vi "Periodic - Drive PID Loop.vi"   [LabVIEW 2012]
uses:
  Globals/Jaguar Commands.vi
  Globals/Robot Jaguars.vi
  Globals/Encoders Global.vi
types:
  T1 = cluster{"proportional gain (Kc)":dbl, "integral time (Ti, min)":dbl, "derivative time (Td, min)":dbl}
  T2 = typedef "WPI_MotorControlDeviceRef.ctl" = cluster{"DeviceStatus":errorcluster, "Type":enum16{"PWM", "CAN"}, "PWM":cluster{"Digital Module":T3, "PWM Channel":T4, "DeadBand":T5}, "CAN":cluster{"Device Number":u8, "Control Mode":T6, "Semaphore":T7, "Max Vout":dbl}, "Invert":bool, "TransformRef":T8, "InvTransformRef":T8}
  T3 = typedef "FPGA_TypedefDigitalModule.ctl" = enum16{"Digital Module 1", "Digital Module 2"}
  T4 = typedef "FPGA_DIOPWMChannel.ctl" = enum8{"PWM 1", "PWM 2", "PWM 3", "PWM 4", "PWM 5", "PWM 6", "PWM 7", "PWM 8", "PWM 9", "PWM 10", "Invalid"}
  T5 = typedef "WPI_PWMDeadband.ctl" = cluster{"Name":string, "maxPositivePwm":i32, "minPositivePwm":i32, "centerPwm":i32, "maxNegativePwm":i32, "minNegativePwm":i32, "angularRange":u16}
  T6 = typedef "WPI_CANJaguar_ControlMode.ctl" = enum8{"Percent VBus", "Current", "Speed", "Position", "Voltage"}
  T7 = typedef "Semaphore RefNum" = refnum<k1>
  T8 = typedef "WPI_PWMTransform_ConPane.ctl" = refnum<vi>
  T9 = cluster{"Front Left Drive":T2, "Front Right Drive":T2, "Rear Left Drive":T2, "Rear Right Drive":T2, "Front Left Steer":T2, "Front Right Steer":T2, "Rear Left Steer":T2, "Rear Right Steer":T2}
  T10 = typedef "WPI_EncoderDevRef.ctl" = cluster{"DevStatus":errorcluster, "EncoderIndex":T11, "CounterIndex":T12, "DistancePerCount":dbl, "Decoding Type":T13}
  T11 = typedef "FPGA_EncoderIdx.ctl" = enum8{"Enc 0", "Enc 1", "Enc 2", "Enc 3", "Invalid"}
  T12 = typedef "FPGA_CounterCtrSystemIndex.ctl" = enum8{"Ctr 0", "Ctr 1", "Ctr 2", "Ctr 3", "Ctr 4", "Ctr 5", "Ctr 6", "Ctr 7", "Invalid"}
  T13 = typedef "WPI_EncoderType.ctl" = enum16{"1x", "2x", "4x"}
  T14 = cluster{"Front Left":T10, "Front Right":T10, "Rear Left":T10, "Rear Right":T10, "Shooter":T10}
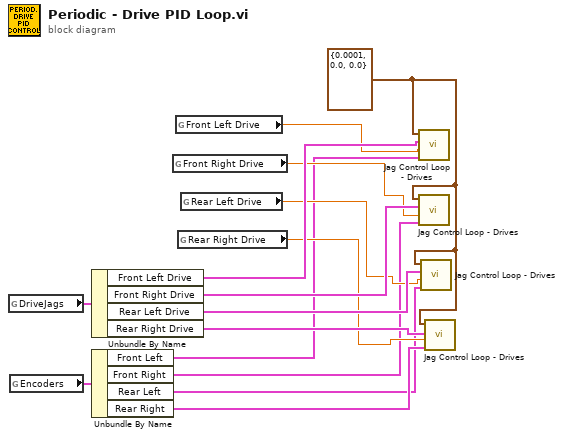
[diagram p0: block diagram]
diagram:
  w14 = T1 {"proportional gain (Kc)"=0.0001, "integral time (Ti, min)"=0.0, "derivative time (Td, min)"=0.0} ("PID gains (Drives)")
  n1 = global read "Robot Jaguars.vi" "DriveJags"() -> (w1:T9)
  n2 = global read "Encoders Global.vi" "Encoders"() -> (w2:T14)
  n3 = Unbundle By Name(w1) -> ("Front Left Drive"=w10:T2, "Front Right Drive"=w11:T2, "Rear Left Drive"=w12:T2, "Rear Right Drive"=w13:T2)
  n4 = Unbundle By Name(w2) -> ("Front Left"=w3:T10, "Front Right"=w4:T10, "Rear Left"=w5:T10, "Rear Right"=w15:T10)
  n5 = global read "Jaguar Commands.vi" "Front Right Drive"() -> (w6:dbl)
  n6 = global read "Jaguar Commands.vi" "Front Left Drive"() -> (w7:dbl)
  n7 = global read "Jaguar Commands.vi" "Rear Right Drive"() -> (w9:dbl)
  n8 = global read "Jaguar Commands.vi" "Rear Left Drive"() -> (w8:dbl)
  n9 = call "Jag Control Loop - Drives.vi"("PID gains"=w14, "MotorControlDevRef"=w10, "Command"=w7, "EncoderDevRef"=w3) -> ()  [unwired: 7 in]
  n10 = call "Jag Control Loop - Drives.vi"("PID gains"=w14, "MotorControlDevRef"=w11, "Command"=w6, "EncoderDevRef"=w4) -> ()  [unwired: 7 in]
  n11 = call "Jag Control Loop - Drives.vi"("PID gains"=w14, "MotorControlDevRef"=w12, "Command"=w8, "EncoderDevRef"=w5) -> ()  [unwired: 7 in]
  n12 = call "Jag Control Loop - Drives.vi"("PID gains"=w14, "MotorControlDevRef"=w13, "Command"=w9, "EncoderDevRef"=w15) -> ()  [unwired: 7 in]
